vi "Close Core.vi"(8 "Error In":errorcluster, 11 "CS++Syslog in":refnum<class "CS++Syslog.lvclass">) -> (0 "Error Out":errorcluster, 3 "CS++Syslog out":refnum<class "CS++Syslog.lvclass">)   [LabVIEW 2014, in "CS++Syslog.lvlib" / "CS++Syslog.lvclass"]
doc: "Close the central message logger client."
uses:
  CS++Syslog.lvclass
  CS++Syslog.lvclass/CS++Syslog.ctl
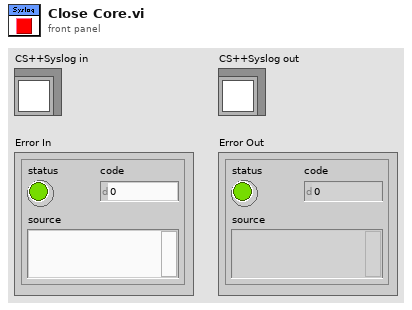
[diagram p1: front panel]
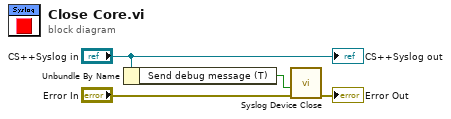
[diagram p0: block diagram]
diagram:
  n1 = Unbundle By Name("CS++Syslog in") -> ("Send debug message (T)"=w1:bool)
  n2 = call <vilib>:"Syslog Device Close.vi"("error in (no error)"="Error In", "Send debug message (T)"=w1) -> ("error out"=→"Error Out":errorcluster)  [unwired: 9 in]
  "CS++Syslog out" <- "CS++Syslog in"
